vi "FGVSavingParameters.vi"(7 "Enum":T1, 8 "error in":errorcluster, 9 "filenameIn":string, 10 "#PicturesSavedIn":u32, 11 "pathIn":path) -> (0 "error out":errorcluster, 1 "filenameOut":string, 2 "#PicturesSavedOut":u32, 3 "pathOut":path)   [LabVIEW 2016]
uses:
  controls/Enum.ctl
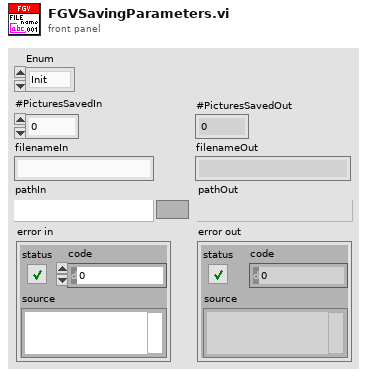
[diagram p1: front panel]
types:
  T1 = typedef "Enum.ctl" = enum16{"Init", "Read", "Write"}
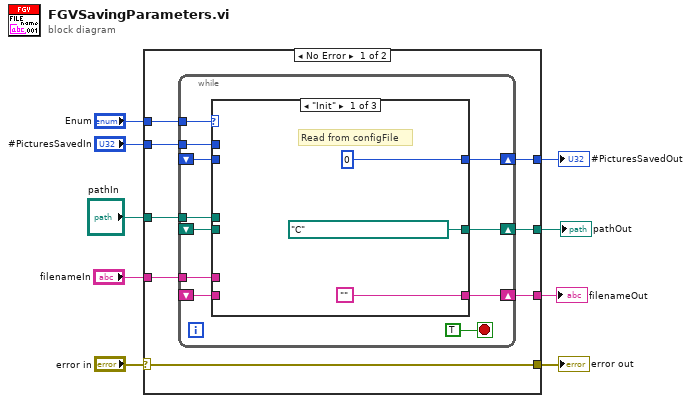
[diagram p0: block diagram]
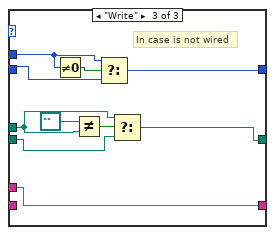
[diagram p3: hidden frame]
diagram:
  n1 = case shown="No Error" "error in" {
    selector: "error in" -> [w16 w48]
    tunnel: "Enum" -> [w17 _]
    tunnel: [w16 w48] -> w8
    tunnel: "pathIn" -> [w15 w47]
    tunnel: [w14 w47] -> w4
    tunnel: [w13 w46] -> w6
    tunnel: "#PicturesSavedIn" -> [w12 w46]
    tunnel: "filenameIn" -> [w11 w45]
    tunnel: [w10 w45] -> w1
    frame No Error {
      n2 = while {
        tunnel: w17 -> [w27]
        tunnel: w15 -> [w26]
        shift-right: [w25] -> w14
        shift-left: _ -> [w24]
        tunnel: w12 -> [w22]
        shift-right: [w23] -> w13
        shift-left: _ -> [w21]
        tunnel: w11 -> [w20]
        shift-right: [w19] -> w10
        shift-left: _ -> [w18]
        stop <- TRUE stop-if-true
        n3 = case shown="\"Init\"" w27 {
          tunnel: w26 -> [_ _ w38]
          tunnel: [path "C:/" ("pathIn") w34 w37] -> w25
          tunnel: w24 -> [_ w34 w39]
          tunnel: [u32 0 w33 w41] -> w23
          tunnel: w22 -> [_ _ w42]
          tunnel: w21 -> [_ w33 w43]
          tunnel: w20 -> [_ _ w35]
          tunnel: ["" w32 w35] -> w19
          tunnel: w18 -> [_ w32 _]
          frame "Init" {
            # "Read from configFile"
          }
          frame "Read", Default {
          }
          frame "Write" {
            # "In case is not wired"
            n4 = Not Equal To 0?(x=w42) -> (x != 0?=w44:bool)
            n5 = Not Equal?(x=path "" ("filenameIn"), y=w38) -> (x != y?=w40:bool)
            n6 = Select(t=w42, s=w44, f=w43) -> (s? t:f=w41:u32)
            n7 = Select(t=w38, s=w40, f=w39) -> (s? t:f=w37:path)
          }
        }
      }
    }
    frame Error {
    }
  }
  "error out" <- w8
  "filenameOut" <- w1
  "#PicturesSavedOut" <- w6
  "pathOut" <- w4
